vi "RT subVI - 2.vi"() -> ()   [LabVIEW 2016]
panel:
  out "reset":bool
  out "slow counter":u16
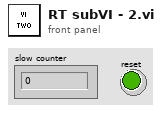
[diagram p1: front panel]
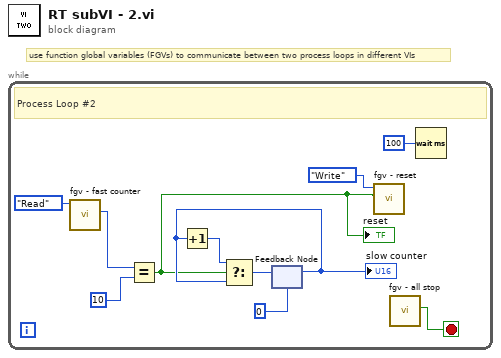
[diagram p0: block diagram]
diagram:
  # "use function global variables (FGVs) to communicate between two process loops in different VIs"
  n1 = while {
    stop <- w1 stop-if-true
    # "Process Loop #2"
    n2 = call "fgv - fast counter.vi"("Operation"=enum16{"Read", "Write"}."Read") -> ("Read Data"=w4:u16)  [unwired: 9 in, 1 out]
    n3 = Equal?(x=w4, y=u16 10) -> (x = y?=w3:bool)
    "reset" <- w3
    n4 = feedback #1(u16 0) -> (w7:u16)
    "slow counter" <- w7
    n5 = Increment(x=w7) -> (x+1=w8:u16)
    n6 = Select(t=w8, s=w3, f=w7) -> (s? t:f=w9:u16)
    n7 = feedback-in #1(w9) -> ()
    n8 = call "fgv - reset.vi"("Write Data (F)"=w3, "Operation"=enum16{"Read", "Write"}."Write") -> ()  [unwired: 8 in, 2 out]
    n9 = call "fgv - all stop.vi"() -> ("Read Data"=w1:bool)  [unwired: 10 in, 1 out]
    n10 = Wait (ms)(milliseconds to wait=u32 100) -> ()  [unwired: 1 out]
  }
